vi "DAQNavi Clear Task.vi"(2 "error in (no error)":errorcluster, 3 "task in":i32) -> (0 "error out":errorcluster)   [LabVIEW 2020]
doc: "Clears the task. Before clearing, this VI aborts the task, if necessary, and releases any resources the task reserved. You can't use a task after you clear it unless you recreate the task."
uses:
  DAQNavi_LV.dll
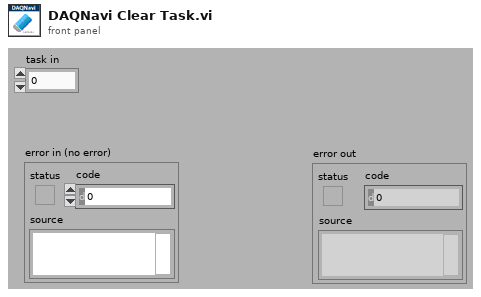
[diagram p1: front panel]
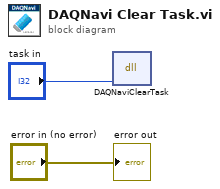
[diagram p0: block diagram]
diagram:
  n1 = dll-call lib="DAQNavi_LV.dll" fn="DAQNaviClearTask"("taskID"="task in") -> ()  [unwired: 4 in, 3 out]
  "error out" <- "error in (no error)"
